vi "Animacion(conSprites)(Bucle).vi"() -> ()   [LabVIEW 2017]
uses:
  <vilib>/picture/picture.llb/Draw True-Color Pixmap.vi
panel:
  in  "delay(ms)":u32=500
  in  "Donde?":cluster{"x":i16, "y":i16}
  out "Mundo":picture
  # "y=214"
  # "125ms"
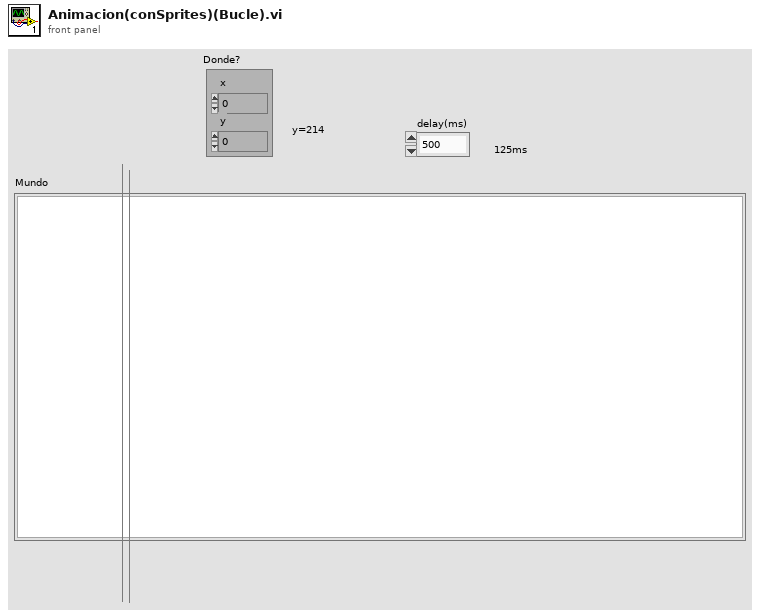
[diagram p1: front panel]
types:
  T1 = typedef "imagedata.ctl" = cluster{"image type":i32, "image depth":i32, "image":u8[], "mask":u8[], "colors":u32[], "Rectangle":cluster{"left":i16, "top":i16, "right":i16, "bottom":i16}}
  T2 = cluster{"left":i16, "top":i16, "right":i16, "bottom":i16}
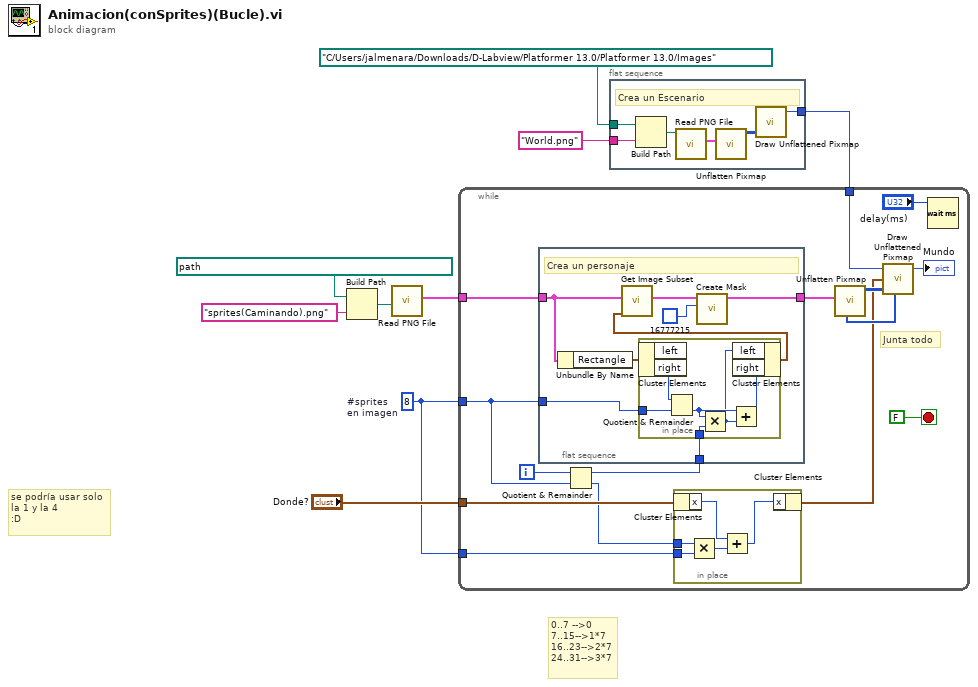
[diagram p0: block diagram]
diagram:
  w1 = i16 8  # #sprites en imagen
  # "se podría usar solo\nla 1 y la 4\n:D"
  # "0..7 -->0\n7..15-->1*7\n16..23-->2*7\n24..31-->3*7"
  n1 = Build Path(base path=path "F:/Prog/LabVIEW/Pruebas/Animación/con sprites" ("path to PNG file"), name or relative path="sprites(Caminando).png" ("format string")) -> (appended path=w6:path)
  n2 = call <vilib>:"Read PNG File.vi"("path to PNG file"=w6) -> ("image data"=w3:T1)  [unwired: 8 in, 2 out]
  n3 = while {
    tunnel: w7 -> [w12]
    tunnel: w3 -> [w22]
    tunnel: "Donde?" -> [w20]
    tunnel: w1 -> [w18]
    tunnel: w1 -> [w16]
    i -> [w19]
    stop <- FALSE stop-if-true
    # "Junta todo"
    n4 = flat-sequence {
      tunnel: w23 -> [w37]
      tunnel: w22 -> [w34]
      tunnel: w18 -> [w35]
      tunnel: [w30] -> w14
      frame #0 {
        # "Crea un personaje"
        n5 = Unbundle By Name(w34) -> ("Rectangle"=w33:T2)
        n6 = in-place {
          in-place-border: w35 -> [w43]
          in-place-border: w37 -> [w41]
          n7 = in-place-cluster #1(w33) -> ("right"=w42:i16)  [unwired: 1 out]
          n8 = Quotient & Remainder(x=w42, y=w43) -> (floor(x/y)=w40:i16)  [unwired: 1 out]
          n9 = Multiply(x=w40, y=w41) -> (x*y=w38:i32)
          n10 = Add(x=w40, y=w38) -> (x+y=w39:i32)
          n11 = in-place-cluster #1("left"=w38, "right"=w39) -> (w36:T2)
        }
        n12 = call <vilib>:"Get Image Subset.vi"("subset rect"=w36, "image data"=w34) -> ("image subset"=w31:T1)  [unwired: 4 in, 1 out]
        n13 = call <vilib>:"Create Mask.vi"("Mask Color (Black)"=u32 16777215 ("Background Color"), "image data"=w31) -> ("image data"=w30:T1)  [unwired: 9 in]
      }
    }
    n14 = Quotient & Remainder(x=w19, y=w18) -> (x-y*floor(x/y)=w23:i32, floor(x/y)=w17:i32)
    n15 = in-place {
      in-place-border: w17 -> [w27]
      in-place-border: w16 -> [w25]
      n16 = in-place-cluster #2(w20) -> ("x"=w29:i16)
      n17 = Multiply(x=w27, y=w25) -> (x*y=w26:i32)
      n18 = Add(x=w29, y=w26) -> (x+y=w28:i32)
      n19 = in-place-cluster #2("x"=w28) -> (w10:cluster{"x":i16, "y":i16})
    }
    n20 = call <vilib>:"Unflatten Pixmap.vi"("image data"=w14) -> ("24-bit pixmap"=w15:u32[][], "mask"=w13:u8[])  [unwired: 4 in, 5 out]
    n21 = call-poly <vilib>:"Draw Unflattened Pixmap.vi"("picture"=w12, "top left point(0, 0)"=w10, "data (RGB format)"=w15, "mask"=w13) -> ("new picture"=→"Mundo":picture)  [unwired: 5 in]
    n22 = Wait (ms)(milliseconds to wait="delay(ms)") -> ()  [unwired: 1 out]
  }
  n23 = flat-sequence {
    tunnel: "World.png" ("format string") -> [w48]
    tunnel: path "C:/Users/jalmenara/Downloads/D-Labview/Platformer 13.0/Platformer 13.0/Images" ("path to PNG file") -> [w47]
    tunnel: [w45] -> w7
    frame #0 {
      # "Crea un Escenario"
      n24 = Build Path(base path=w47, name or relative path=w48) -> (appended path=w46:path)
      n25 = call <vilib>:"Read PNG File.vi"("path to PNG file"=w46) -> ("image data"=w49:T1)  [unwired: 8 in, 2 out]
      n26 = call <vilib>:"Unflatten Pixmap.vi"("image data"=w49) -> ("24-bit pixmap"=w44:u32[][])  [unwired: 4 in, 6 out]
      n27 = call-poly <vilib>:"Draw Unflattened Pixmap.vi"("data (RGB format)"=w44) -> ("new picture"=w45:picture)  [unwired: 8 in]
    }
  }
